vi "myRIO v1.0 Write DMA.vi"   [LabVIEW 2021]
uses:
  <vilib>/myRIO/Common/Instrument Driver Framework/Utilities/typedefs/FPGA Ref Manager Action Enum.ctl
  <vilib>/Platform/TimedLoop/XDataNode/timing_clust.ctl
  <vilib>/Platform/TimedLoop/XDataNode/nitl_modes.ctl
  <vilib>/Platform/TimedLoop/XDataNode/wakeup.ctl
  <vilib>/myRIO/Common/Instrument Driver Framework/myRIO v1.0/AO Block/typedefs/AO Block Channels FPGA Reference.ctl
  <vilib>/myRIO/Common/Instrument Driver Framework/myRIO v1.0/AudioOut Block/typedefs/AudioOut Block Channels FPGA Reference.ctl
  <vilib>/myRIO/Common/Instrument Driver Framework/myRIO v1.0/DO Block/typedefs/DO Block FPGA Reference.ctl
  <vilib>/Utility/error.llb/Error Cluster From Error Code.vi
  <vilib>/RVI Host/nirviSupport.llb/nirviErrorClusterFromErrorCode.vi
  <vilib>/rvi/errors/niLvFpgaAdjustHostInterfaceError.vi
  <vilib>/platform/TimedLoop/XDataNode/XDataNode.xnode
  <vilib>/rvi/interface/nirviMethod/nirviMethod.xnode
  <vilib>/myRIO/Common/Instrument Driver Framework/Utilities/typedefs/Generic FPGA Reference.ctl
  <vilib>/rvi/interface/nirviReadWriteControl/nirviReadWriteControl.xnode
  NiFpgaLv.dll
  <vilib>/rvi/interface/Simulation/niFpgaSimulationCallBeginRW.vi
  <vilib>/FPGAPlugInAG/Dynamic/niLvFpga_WriteFifo_Dynamic.vi
  <vilib>/rvi/errors/niLvFpgaMergeErrorWithErrorCode.vi
  <vilib>/Platform/TimedLoop/XDataNode/XDNodeRunTimeDep.lvlib
  <vilib>/rvi/interface/nirviMethod/StockFPGA_InlinedMethodWaitForMultipleIRQ.vi
  <vilib>/FPGAPlugInAG/Dynamic/niLvFpga_WaitOnIrq_Dynamic.vi
  <vilib>/FPGAPlugInAG/Dynamic/niLvFpga_AcknowledgeIrq_Dynamic.vi
panel:
  # "This VI waits for the IRQ from FPGA. If FPGA DMA buffer is empty, it reads from \nthe resource manager which stores the data and configuration to be written to the FPGA\nand writes to the FPGA.\nAO Block, AudioOut Block and DO Block all use this VI to send data.\nThis VI is called Asynchronously in the myRIO v1.1/v1.2 Open Throughput * Block.vi."
types:
  T1 = typedef "FPGA Ref Manager Action Enum.ctl" = enum16{"Get", "Set", "Reset"}
  T2 = typedef "Generic FPGA Reference.ctl" = refnum<k20>
  T3 = typedef "XDNodeRunTimeDep.lvlib/timing_clust.ctl" = cluster{"Expected End [f-1]":u64, "Actual End [f-1]":u64, "Finished Late? [f-1]":bool, "Expected End [i-1]":u64, "Actual End [i-1]":u64, "Finished Late? [i-1]":bool, "Expected Start [i]":u64, "Actual Start [i]":u64, "Expected Start [f]":u64, "Actual Start [f]":u64, "Source Name":string, "Structure Name":string, "Period":i64, "Deadline":i64, "Offset":i64, "Start":i64, "Priority":i32, "Timeout":i32, "Mode":T4, "Wakeup Reason":T5, "Error":errorcluster, "Source Type":string, "Secondary Source Type":string, "Global End Time":u64, "Global Start Time":u64, "Frame Duration":u64, "Iteration Duration":u64, "Assigned CPU":i32, "I/O Scan Engine Mode":u32}
  T4 = typedef "XDNodeRunTimeDep.lvlib/nitl_modes.ctl" = enum32{"No Change", "Process missed periods, maintain original phase", "Discard missed periods, maintain original phase", "Process missed periods, ignore original phase", "Discard missed periods, ignore original phase"}
  T5 = typedef "XDNodeRunTimeDep.lvlib/wakeup.ctl" = enum32{"Normal", "Aborted", "Asynchronous wakeup", "Timing source error", "Timed loop error", "Timeout"}
  T6 = enum16{"A/AO0 Block", "AudioOut Block", "A/DO1 Block", "None"}
  T7 = typedef "AO Block Channels FPGA Reference.ctl" = refnum<k20>
  T8 = typedef "AO Block Configuration.ctl" = cluster{"Wait Until Done?":bool, "AO FIFO Sample Rate(ticks)":u32, "Occurrence Handler ":refnum<k4>, "Analog data reference":refnum<data-value>}
  T9 = typedef "AudioOut Block Channels FPGA Reference.ctl" = refnum<k20>
  T10 = typedef "AudioOut Block Configuration.ctl" = cluster{"Wait Until Done?":bool, "AudioOut FIFO Sample Rate(ticks)":u32, "Occurrence Handler":refnum<k4>, "Audio data reference":refnum<data-value>}
  T11 = typedef "DO Block FPGA Reference.ctl" = refnum<k20>
  T12 = typedef "DO Block Configuration.ctl" = cluster{"Wait Until Done?":bool, "DO FIFO Clock Divisor":u16, "Occurrence Handler":refnum<k4>, "Digital data reference":refnum<data-value>}
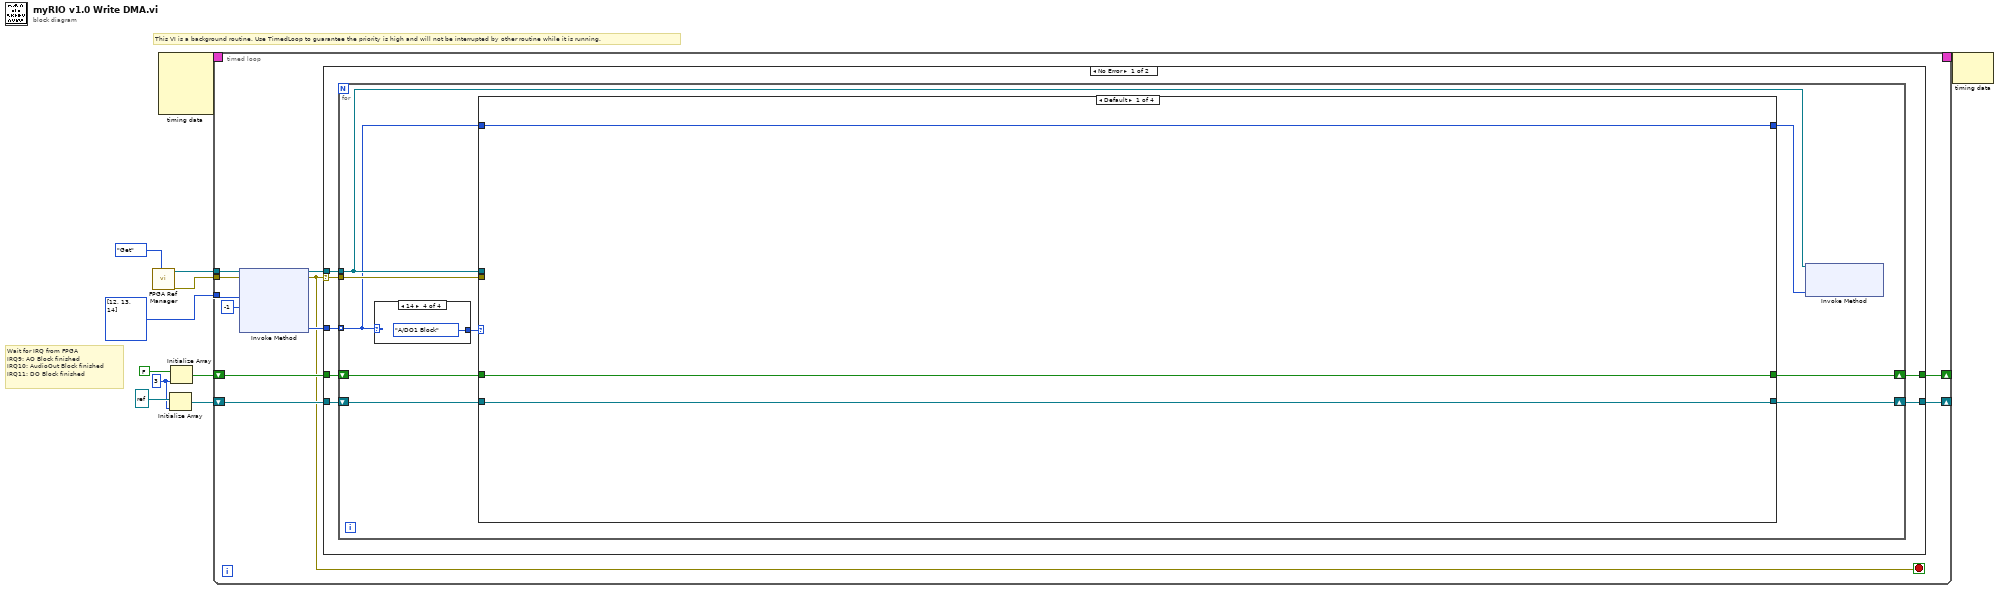
[diagram p0: block diagram]
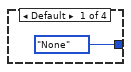
[diagram p2: hidden frame]
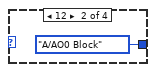
[diagram p3: hidden frame]
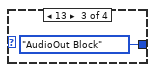
[diagram p4: hidden frame]
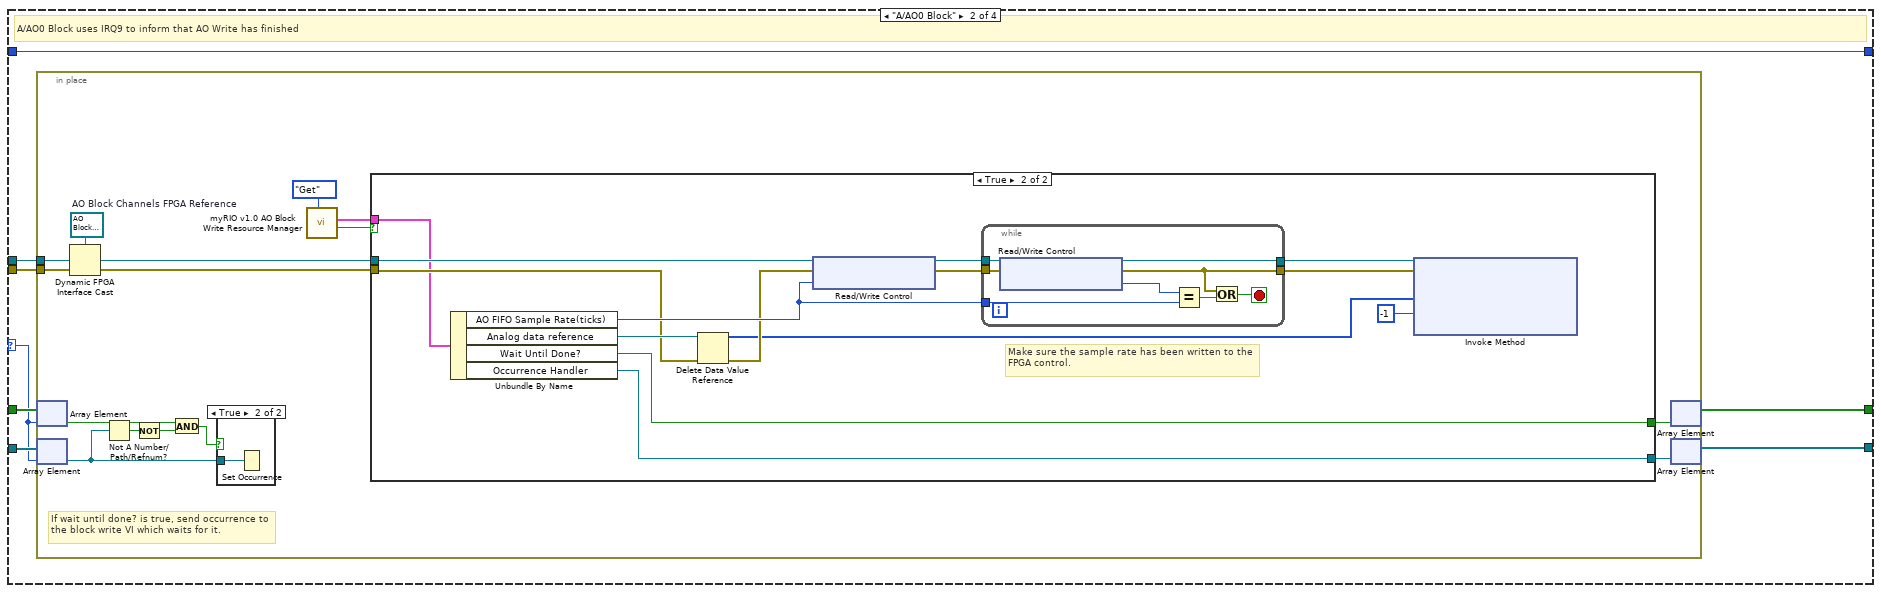
[diagram p5: hidden frame]
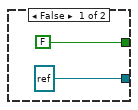
[diagram p6: hidden frame]
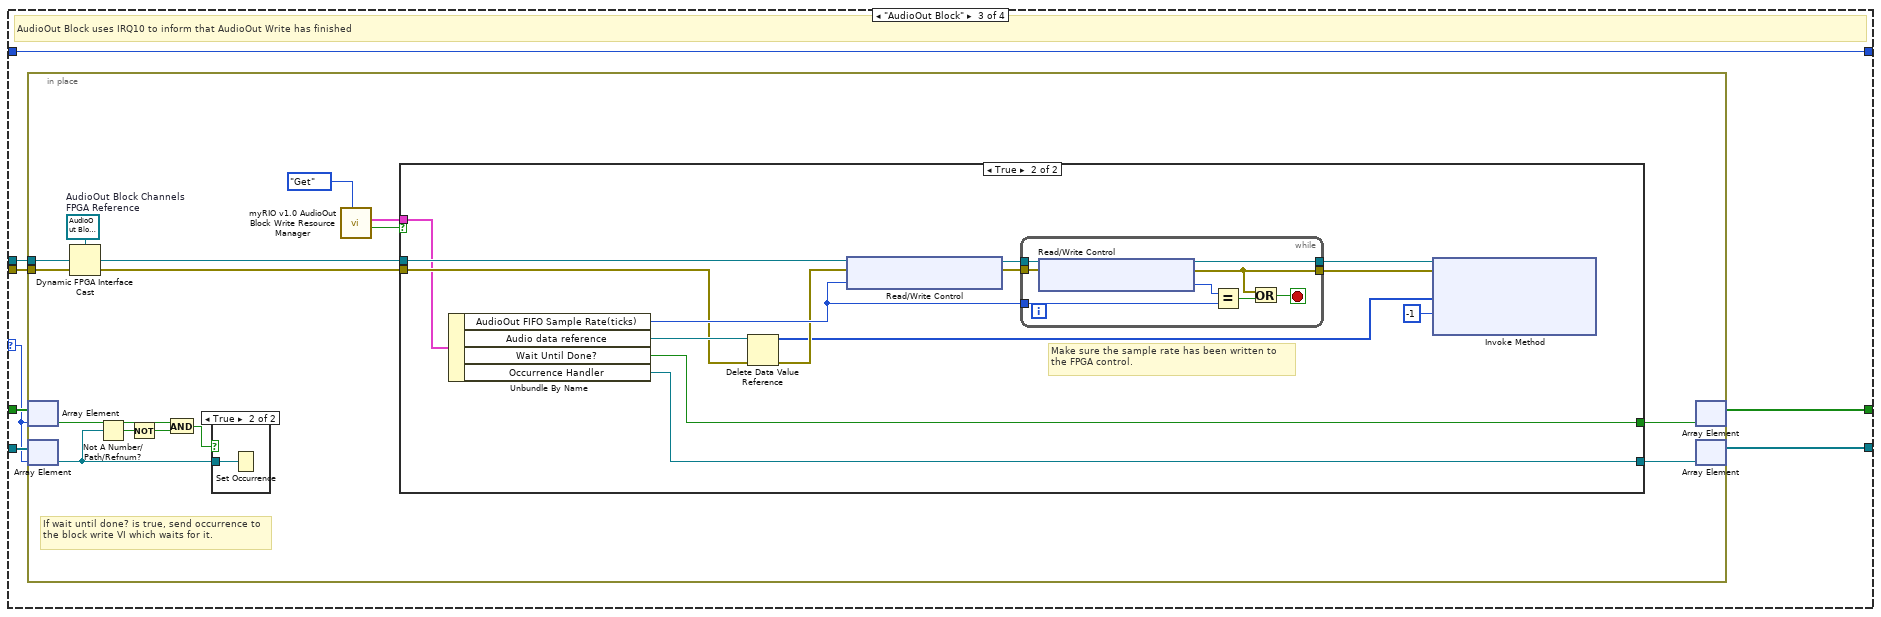
[diagram p8: hidden frame]
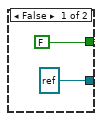
[diagram p9: hidden frame]
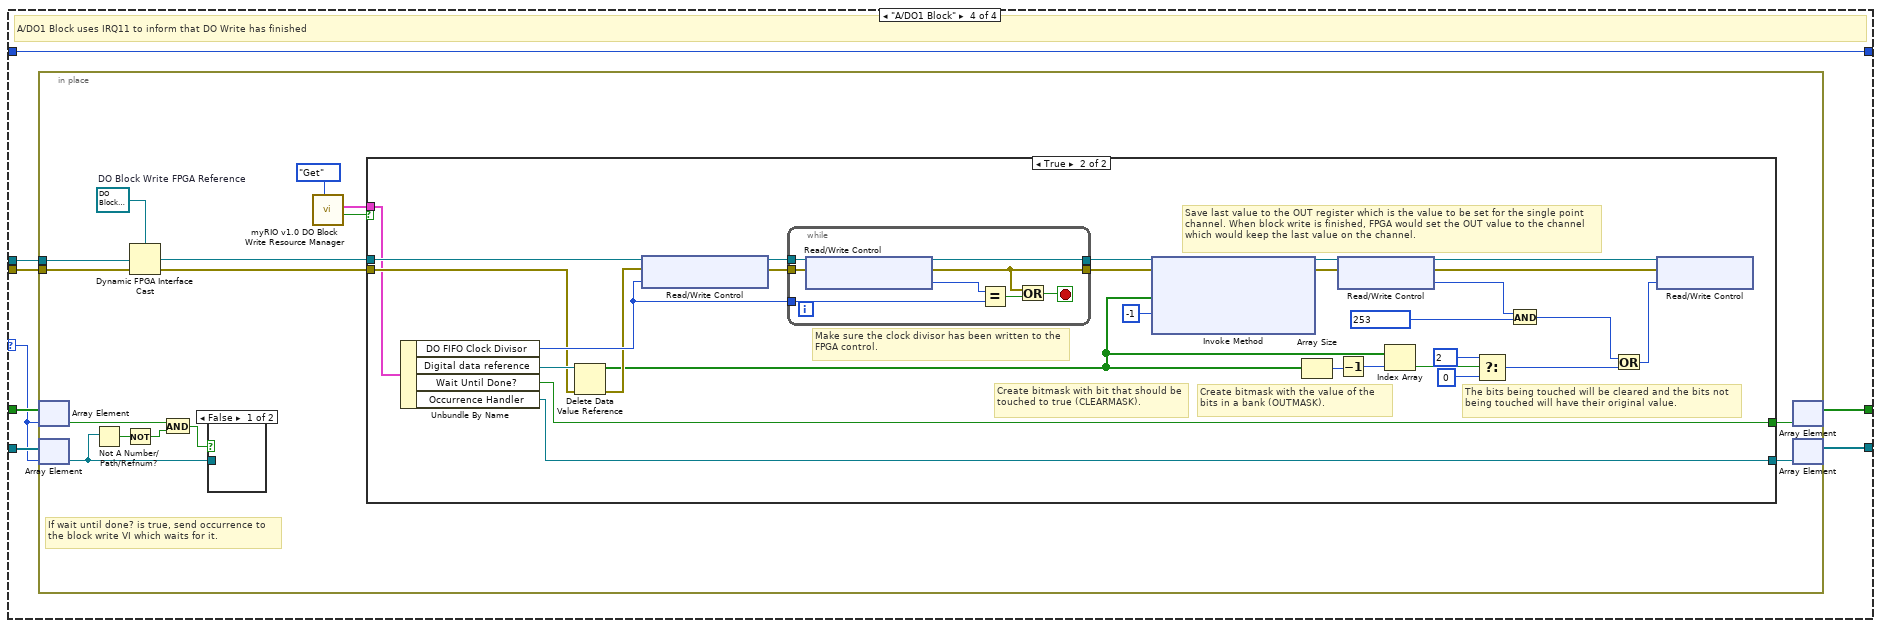
[diagram p11: hidden frame]
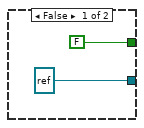
[diagram p12: hidden frame]
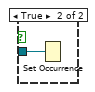
[diagram p13: hidden frame]
diagram:
  w3 = 3 ("dimension size")
  # "This VI is a background routine. Use TimedLoop to guarantee the priority is high and will not be interrupted by other routine while it is running."
  # "Wait for IRQ from FPGA\nIRQ9: AO Block finished\nIRQ10: AudioOut Block finished\nIRQ11: DO Block finished"
  n1 = call <vilib>:"FPGA Ref Manager.vi"("Action"=FPGA_Ref_Manager_Action_Enum."Get") -> ("error out"=w10:errorcluster, "Generic FPGA Reference out"=w8:T2)  [unwired: 8 in]
  n2 = node-c288() -> (w2:T3)  [unwired: 4 in]
  n3 = Initialize Array(refnum<k4> refnum ("Occurrence Handler"), w3) -> (w6:refnum<k4>[])
  n4 = Initialize Array(FALSE, w3) -> (w4:bool[])
  n5 = timed-loop {
    tunnel: w10 -> [w22]
    tunnel: i32[] [12, 13, 14] -> [w21]
    tunnel: w8 -> [w20]
    shift-right: [w13] -> _
    shift-left: w4 -> [w18]
    shift-right: [w12] -> _
    shift-left: w6 -> [w19]
    timing: w2 -> [_]
    timing-out: [_] -> w1
    stop <- w14 stop-if-true
    n6 = xnode "Invoke Method"("FPGA VI Reference In"=w20, "error in"=w22, "IRQ Number(s)"=w21, "Timeout (ms)"=-1) -> ("FPGA VI Reference Out"=w16:T2, "error out"=w14:errorcluster, "IRQ(s) Asserted"=w15:i32[])  [unwired: 1 out]
    n7 = case shown="No Error" w14 {
      selector: w14 -> [w23 _]
      tunnel: w16 -> [w29 _]
      tunnel: w15 -> [w28 _]
      tunnel: [w27 w202] -> w13
      tunnel: [w26 w201] -> w12
      tunnel: w18 -> [w25 w202]
      tunnel: w19 -> [w24 w201]
      frame No Error {
        n8 = for {
          tunnel: w29 -> [w32]
          tunnel: w28 -> [w31] mode=indexing
          tunnel: w23 -> [w34]
          shift-right: [w38] -> w27
          shift-left: w25 -> [w36]
          shift-right: [w37] -> w26
          shift-left: w24 -> [w35]
          n9 = case shown="14" w31 {
            tunnel: [T6."None" T6."A/AO0 Block" T6."AudioOut Block" T6."A/DO1 Block"] -> w33
            frame Default {
            }
            frame 12 {
            }
            frame 13 {
            }
            frame 14 {
            }
          }
          n10 = case shown="Default" w33 {
            selector: w33 -> [_ w47 w94 w141]
            tunnel: w32 -> [_ w51 w98 w145]
            tunnel: [w45 w49 w97 w143] -> w38
            tunnel: [w44 w48 w96 w142] -> w37
            tunnel: w36 -> [w45 w53 w100 w147]
            tunnel: w35 -> [w44 w52 w99 w146]
            tunnel: w34 -> [_ w50 w95 w144]
            tunnel: w31 -> [w43 w46 w93 w140]
            tunnel: [w43 w46 w93 w140] -> w30
            frame Default {
            }
            frame "A/AO0 Block" {
              # "A/AO0 Block uses IRQ9 to inform that AO Write has finished"
              n11 = in-place {
                in-place-border: w51 -> [w60]
                in-place-border: w50 -> [w59]
                w61 = T7 refnum  # AO Block Channels FPGA Reference
                # "If wait until done? is true, send occurrence to the block write VI which waits for it."
                n12 = in-place-array #1(w53, w47) -> (w64:bool)
                n13 = in-place-array #2(w52, w47) -> (w58:refnum<k4>)
                n14 = Dynamic FPGA Interface Cast(Session In=w61, Type=w60) -> (Session Out=w57:T7)
                n15 = Not A Number/Path/Refnum?(number/path/refnum=w58) -> (NaN/Path/Refnum?=w67:bool)
                n16 = Not(x=w67) -> (.not. x?=w65:bool)
                n17 = And(x=w64, y=w65) -> (x .and. y?=w66:bool)
                n18 = case shown="True" w66 {
                  tunnel: w58 -> [_ w92]
                  frame False {
                  }
                  frame True {
                    n19 = Set Occurrence(w92) -> ()
                  }
                }
                n20 = call <vilib>:"myRIO v1.0 AO Block Write Resource Manager.vi"("Action"=enum16{"Get", "Set"}."Get") -> ("Action Succeeds"=w55:bool, "AO Resource Out"=w54:T8)  [unwired: 9 in]
                n21 = case shown="True" w55 {
                  tunnel: w57 -> [_ w83]
                  tunnel: w54 -> [_ w70]
                  tunnel: [FALSE ("Wait Until Done?") w76] -> w63
                  tunnel: [refnum<k4> refnum ("Occurrence Handler") w75] -> w62
                  tunnel: w59 -> [_ w73]
                  frame False {
                  }
                  frame True {
                    # "Make sure the sample rate has been written to the FPGA control."
                    n22 = Unbundle By Name(w70) -> ("AO FIFO Sample Rate(ticks)"=w77:u32, "Analog data reference"=w74:refnum<data-value>, "Wait Until Done?"=w76:bool, "Occurrence Handler"=w75:refnum<k4>)
                    n23 = Delete Data Value Reference(data value reference=w74, error in=w73) -> (data value=w71:u16[], error out=w72:errorcluster)
                    n24 = xnode "Read/Write Control"("FPGA VI Reference In"=w83, "error in"=w72, "AO.A_0.SampleRate"=w77) -> ("FPGA VI Reference Out"=w82:T7, "error out"=w81:errorcluster)
                    n25 = while {
                      tunnel: w82 -> [w91]
                      tunnel: [w90] -> w80
                      tunnel: [w85] -> w79
                      tunnel: w81 -> [w89]
                      tunnel: w77 -> [w88]
                      stop <- w84 stop-if-true
                      n26 = xnode "Read/Write Control"("FPGA VI Reference In"=w91, "error in"=w89) -> ("FPGA VI Reference Out"=w90:T7, "error out"=w85:errorcluster, "AO.A_0.SampleRate"=w87:u32)
                      n27 = Equal?(x=w87, y=w88) -> (x = y?=w86:bool)
                      n28 = Or(x=w85, y=w86) -> (x .or. y?=w84:bool)
                    }
                    n29 = xnode "Invoke Method"("FPGA VI Reference In"=w80, "error in"=w79, "Data"=w71, "Timeout (ms)"=-1) -> ()  [unwired: 3 out]
                  }
                }
                n30 = in-place-array #1(w63) -> (w49:bool[])  [unwired: 1 out]
                n31 = in-place-array #2(w62) -> (w48:refnum<k4>[])  [unwired: 1 out]
              }
            }
            frame "AudioOut Block" {
              # "AudioOut Block uses IRQ10 to inform that AudioOut Write has finished"
              n32 = in-place {
                in-place-border: w98 -> [w106]
                in-place-border: w95 -> [w105]
                w107 = T9 refnum  # AudioOut Block Channels FPGA Reference
                # "If wait until done? is true, send occurrence to the block write VI which waits for it."
                n33 = in-place-array #3(w100, w94) -> (w111:bool)
                n34 = in-place-array #4(w99, w94) -> (w110:refnum<k4>)
                n35 = Dynamic FPGA Interface Cast(Session In=w107, Type=w106) -> (Session Out=w104:T9)
                n36 = Not A Number/Path/Refnum?(number/path/refnum=w110) -> (NaN/Path/Refnum?=w114:bool)
                n37 = Not(x=w114) -> (.not. x?=w112:bool)
                n38 = And(x=w111, y=w112) -> (x .and. y?=w113:bool)
                n39 = case shown="True" w113 {
                  tunnel: w110 -> [_ w139]
                  frame False {
                  }
                  frame True {
                    n40 = Set Occurrence(w139) -> ()
                  }
                }
                n41 = call <vilib>:"myRIO v1.0 AudioOut Block Write Resource Manager.vi"("Action"=enum16{"Get", "Set"}."Get") -> ("Action Succeeds"=w102:bool, "AudioOut Resource Out"=w101:T10)  [unwired: 9 in]
                n42 = case shown="True" w102 {
                  tunnel: w104 -> [_ w130]
                  tunnel: [FALSE ("Wait Until Done?") w123] -> w109
                  tunnel: [refnum<k4> refnum ("Occurrence Handler") w122] -> w108
                  tunnel: w105 -> [_ w120]
                  tunnel: w101 -> [_ w117]
                  frame False {
                  }
                  frame True {
                    # "Make sure the sample rate has been written to the FPGA control."
                    n43 = Unbundle By Name(w117) -> ("AudioOut FIFO Sample Rate(ticks)"=w124:u32, "Audio data reference"=w121:refnum<data-value>, "Wait Until Done?"=w123:bool, "Occurrence Handler"=w122:refnum<k4>)
                    n44 = Delete Data Value Reference(data value reference=w121, error in=w120) -> (data value=w118:u32[], error out=w119:errorcluster)
                    n45 = xnode "Read/Write Control"("FPGA VI Reference In"=w130, "error in"=w119, "AO.AudioOut.SampleRate"=w124) -> ("FPGA VI Reference Out"=w129:T9, "error out"=w128:errorcluster)
                    n46 = while {
                      tunnel: w129 -> [w138]
                      tunnel: [w137] -> w127
                      tunnel: [w133] -> w126
                      tunnel: w128 -> [w136]
                      tunnel: w124 -> [w135]
                      stop <- w132 stop-if-true
                      n47 = xnode "Read/Write Control"("FPGA VI Reference In"=w138, "error in"=w136) -> ("FPGA VI Reference Out"=w137:T9, "error out"=w133:errorcluster, "AO.AudioOut.SampleRate"=w131:u32)
                      n48 = Equal?(x=w131, y=w135) -> (x = y?=w134:bool)
                      n49 = Or(x=w133, y=w134) -> (x .or. y?=w132:bool)
                    }
                    n50 = xnode "Invoke Method"("FPGA VI Reference In"=w127, "error in"=w126, "Data"=w118, "Timeout (ms)"=-1) -> ()  [unwired: 3 out]
                  }
                }
                n51 = in-place-array #3(w109) -> (w97:bool[])  [unwired: 1 out]
                n52 = in-place-array #4(w108) -> (w96:refnum<k4>[])  [unwired: 1 out]
              }
            }
            frame "A/DO1 Block" {
              # "A/DO1 Block uses IRQ11 to inform that DO Write has finished"
              n53 = in-place {
                in-place-border: w145 -> [w154]
                in-place-border: w144 -> [w152]
                w153 = T11 refnum  # DO Block Write FPGA Reference
                # "If wait until done? is true, send occurrence to the block write VI which waits for it."
                n54 = in-place-array #5(w147, w141) -> (w158:bool)
                n55 = in-place-array #6(w146, w141) -> (w157:refnum<k4>)
                n56 = Not A Number/Path/Refnum?(number/path/refnum=w157) -> (NaN/Path/Refnum?=w161:bool)
                n57 = Not(x=w161) -> (.not. x?=w159:bool)
                n58 = Dynamic FPGA Interface Cast(Session In=w153, Type=w154) -> (Session Out=w151:T11)
                n59 = And(x=w158, y=w159) -> (x .and. y?=w160:bool)
                n60 = case shown="False" w160 {
                  tunnel: w157 -> [_ w200]
                  frame False {
                  }
                  frame True {
                    n61 = Set Occurrence(w200) -> ()
                  }
                }
                n62 = call <vilib>:"myRIO v1.0 DO Block Write Resource Manager.vi"("Action"=enum16{"Get", "Set"}."Get") -> ("Action Succeeds"=w149:bool, "DO Resource Out"=w148:T12)  [unwired: 9 in]
                n63 = case shown="True" w149 {
                  tunnel: w151 -> [_ w191]
                  tunnel: [FALSE ("Wait Until Done?") w186] -> w156
                  tunnel: [refnum<k4> refnum ("Occurrence Handler") w185] -> w155
                  tunnel: w152 -> [_ w171]
                  tunnel: w148 -> [_ w164]
                  frame False {
                  }
                  frame True {
                    # "Save last value to the OUT register which is the value to be set for the single point channel. When block write is finished, FPGA would set the OUT value to the channel which would keep the last value on the channel."
                    # "Create bitmask with bit that should be touched to true (CLEARMASK)."
                    # "The bits being touched will be cleared and the bits not being touched will have their original value."
                    # "Create bitmask with the value of the bits in a bank (OUTMASK)."
                    # "Make sure the clock divisor has been written to the FPGA control."
                    n64 = Unbundle By Name(w164) -> ("DO FIFO Clock Divisor"=w187:u16, "Digital data reference"=w172:refnum<data-value>, "Wait Until Done?"=w186:bool, "Occurrence Handler"=w185:refnum<k4>)
                    n65 = Delete Data Value Reference(data value reference=w172, error in=w171) -> (data value=w168:bool[], error out=w170:errorcluster)
                    n66 = xnode "Read/Write Control"("FPGA VI Reference In"=w191, "error in"=w170, "DO.A_1.ClockDivisor"=w187) -> ("FPGA VI Reference Out"=w190:T11, "error out"=w189:errorcluster)
                    n67 = while {
                      tunnel: w190 -> [w199]
                      tunnel: [w198] -> w174
                      tunnel: [w194] -> w173
                      tunnel: w189 -> [w197]
                      tunnel: w187 -> [w196]
                      stop <- w193 stop-if-true
                      n68 = xnode "Read/Write Control"("FPGA VI Reference In"=w199, "error in"=w197) -> ("FPGA VI Reference Out"=w198:T11, "error out"=w194:errorcluster, "DO.A_1.ClockDivisor"=w192:u16)
                      n69 = Equal?(x=w192, y=w196) -> (x = y?=w195:bool)
                      n70 = Or(x=w194, y=w195) -> (x .or. y?=w193:bool)
                    }
                    n71 = xnode "Invoke Method"("FPGA VI Reference In"=w174, "error in"=w173, "Data"=w168, "Timeout (ms)"=-1) -> ("FPGA VI Reference Out"=w166:T11, "error out"=w165:errorcluster)  [unwired: 1 out]
                    n72 = Array Size(array=w168) -> (size(s)=w169:i32)
                    n73 = xnode "Read/Write Control"("FPGA VI Reference In"=w166, "error in"=w165) -> ("FPGA VI Reference Out"=w183:T11, "error out"=w184:errorcluster, "DIO.A_7:0.OUT"=w178:u8)
                    n74 = Decrement(x=w169) -> (x-1=w176:i32)
                    n75 = Index Array(array=w168, index=w176) -> (element=w167:bool)
                    n76 = Select(t=u8 2 ("y"), s=w167, f=u8 0 ("y")) -> (s? t:f=w182:u8)
                    n77 = And(x=w178, y=u8 253) -> (x .and. y?=w180:u8)
                    n78 = Or(x=w180, y=w182) -> (x .or. y?=w177:u8)
                    n79 = xnode "Read/Write Control"("FPGA VI Reference In"=w183, "error in"=w184, "DIO.A_7:0.OUT"=w177) -> ()  [unwired: 2 out]
                  }
                }
                n80 = in-place-array #5(w156) -> (w143:bool[])  [unwired: 1 out]
                n81 = in-place-array #6(w155) -> (w142:refnum<k4>[])  [unwired: 1 out]
              }
            }
          }
          n82 = xnode "Invoke Method"("FPGA VI Reference In"=w32, "IRQ Number(s)"=w30) -> ()  [unwired: 1 in, 2 out]
        }
      }
      frame Error {
      }
    }
  }
  n83 = node-c288(w1) -> ()  [unwired: 1 out]
